vi "niWLAN - OPPO - 80211abgnGeneration(ref).vi"(0 "Rx Measurements Settings":T2 {"DSSS Data Rate (Mbps)" items=["1", "2", "5.5 CCK", "5.5 PBCC", "11 CCK", "11 PBCC", "22", "33"]; "OFDM Data Rate (Mbps)" items=["6", "9", "12", "18", "24", "36", "48", "54"]; "80211n PLCP Frame Format" items=["Mixed Format", "Greenfield Format"]; "Standard" items=["80211A/G/J/P OFDM", "80211B/G DSSS", "80211G DSSSOFDM", "80211N MIMOOFDM", "80211AC MIMOOFDM"]}, 5 "Without ACK ?":bool, 7 "Address String":string="00:90:4C:C5:12:38", 11 "error in":errorcluster) -> (4 "Cluster":T1, 15 "error out":errorcluster)   [LabVIEW 2010]
uses:
  <libdir>/resource/objmgr/niWLANGeneration.rc
  <vilib>/RF Toolkits/WLAN/generation/niWLANG Create Multiple Channel Waveform (IQ Complex Cluster).vi
  <vilib>/RF Toolkits/WLAN/generation/niWLANG Create Single Channel Waveform (IQ Complex Cluster).vi
  <vilib>/RF Toolkits/WLAN/generation/controls/wlanG version control.ctl
  TV/RW/Includes/WLAN - TV - RW - INC - Rx_PER_Wfm_Settings.ctl
panel:
  in  "Boolean":bool
  in  "Idle Time (With Ack)":dbl
  in  "file path":path
  # "Hardware Configuration"
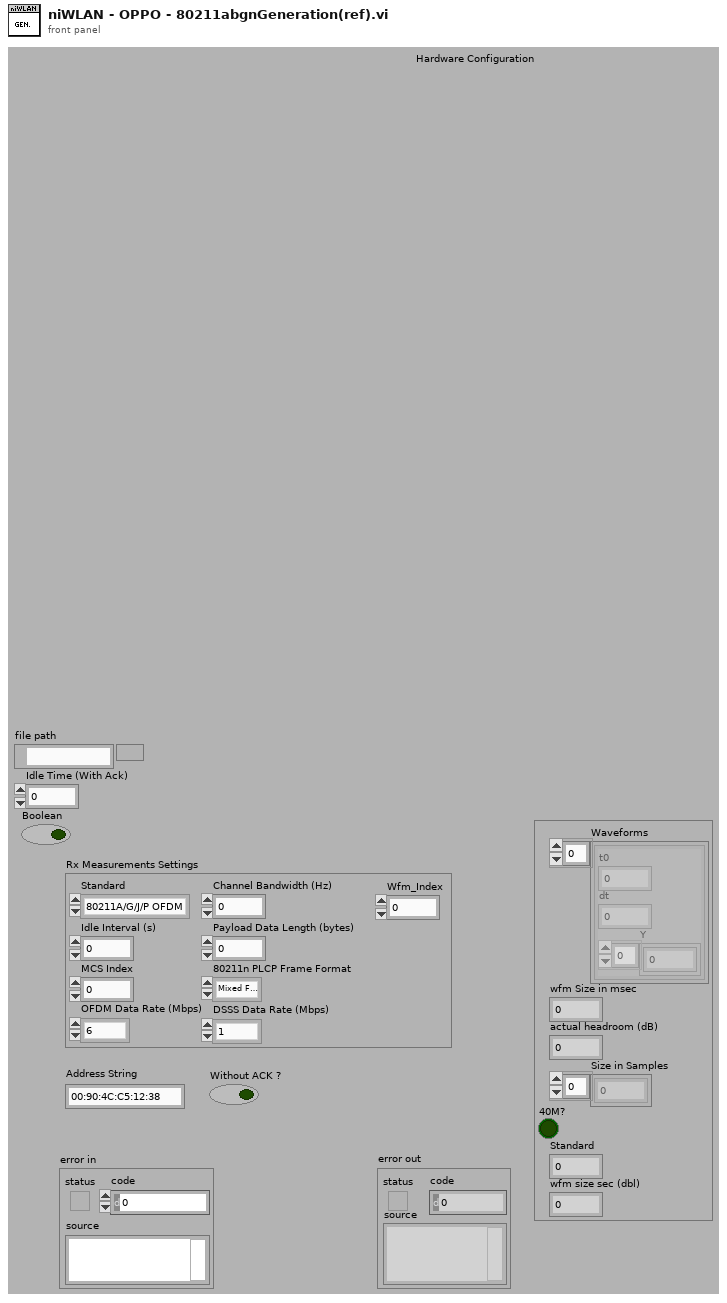
[diagram p1: front panel]
types:
  T1 = cluster{"Waveforms":cluster{"t0":dbl, "dt":dbl, "Y":cdb[]}[], "wfm Size in msec":i32, "actual headroom (dB)":dbl, "Size in Samples":i32[], "40M?":bool, "Standard ":i32, "wfm size sec (dbl)":dbl}
  T2 = typedef "WLAN - TV - RW - INC - Rx_PER_Wfm_Settings.ctl" = cluster{"Standard":i32, "Channel Bandwidth (Hz)":dbl, "Idle Interval (s)":dbl, "MCS Index":i32, "80211n PLCP Frame Format":i32, "Payload Data Length (bytes)":i32, "OFDM Data Rate (Mbps)":i32, "DSSS Data Rate (Mbps)":i32, "Wfm_Index":i32}
  T3 = typedef "wlanG version control.ctl" = i32
  T4 = typedef "wlanv1_generation refnum.ctl" = refnum<k20>
  T5 = typedef "wlanv1_Generation Refnum.ctl" = refnum<k20>
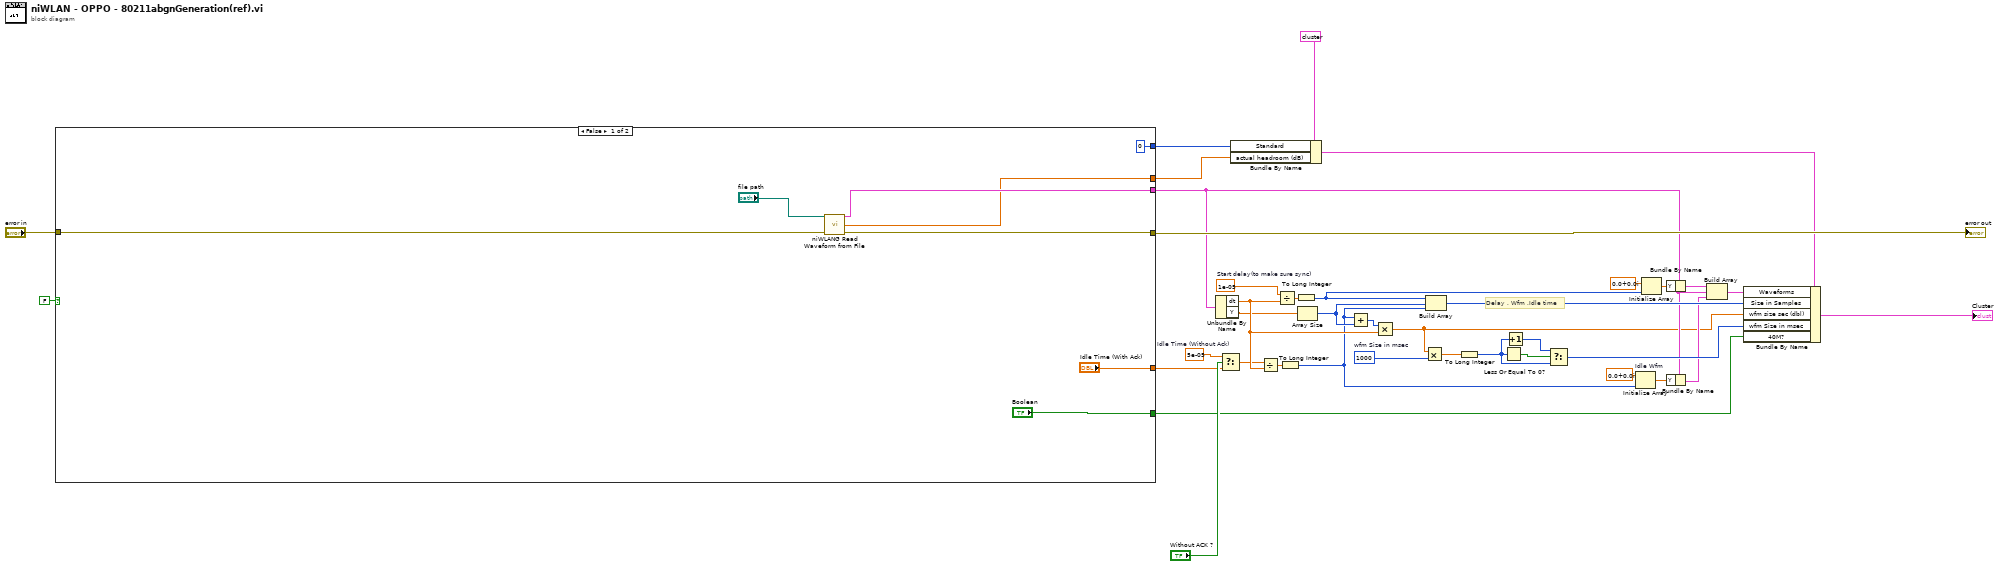
[diagram p0: block diagram]
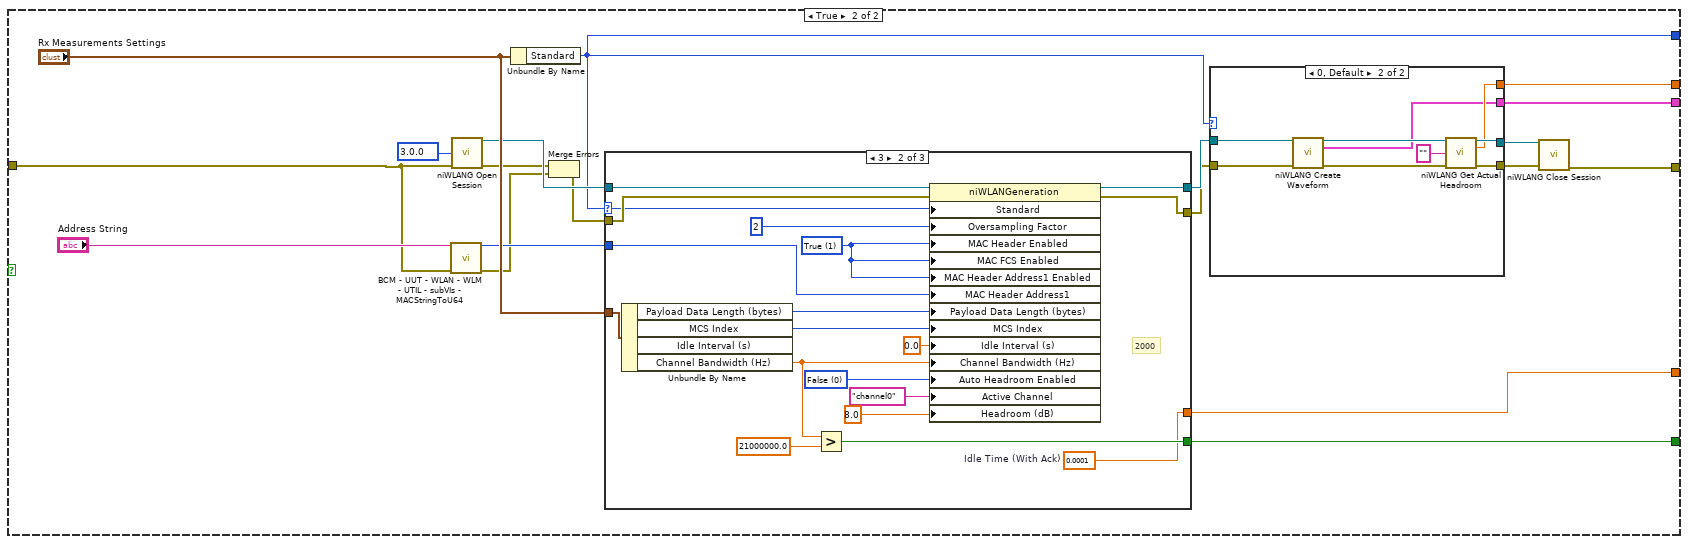
[diagram p2: hidden frame]
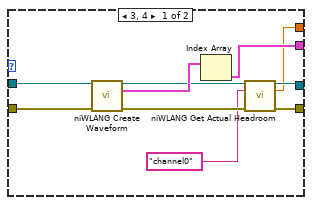
[diagram p3: hidden frame]
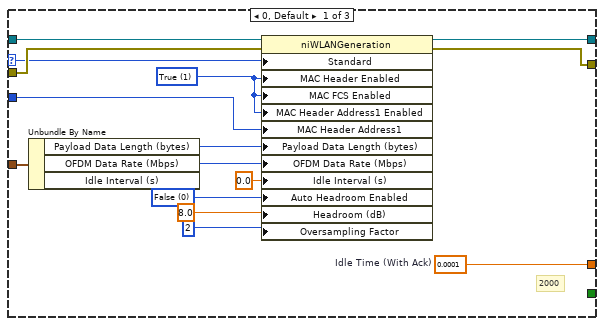
[diagram p4: hidden frame]
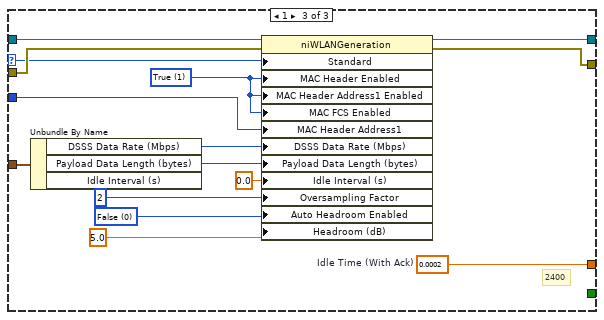
[diagram p5: hidden frame]
diagram:
  w16 = 1e-05  # Start delay(to make sure sync)
  w6 = 5e-05  # Idle Time (Without Ack)
  w15 = 1000  # wfm Size in msec
  # "Delay , Wfm ,Idle time"
  n1 = case shown="False" FALSE {
    tunnel: [w46 w64] -> w38
    tunnel: ["Boolean" w52] -> w25
    tunnel: [w45 w51] -> w18
    tunnel: [0 ("Standard") w50] -> w10
    tunnel: [w44 w49] -> w8
    tunnel: ["Idle Time (With Ack)" w48] -> w4
    tunnel: "error in" -> [w43 w47]
    frame False {
      n2 = call <vilib>:"niWLANG Read Waveform from File.vi"("file path"="file path", "error in"=w43) -> ("waveform"=w45:cluster{"t0":dbl, "dt":dbl, "Y":cdb[]}, "headroom (dB)"=w44:dbl, "error out"=w46:errorcluster)  [unwired: 9 in, 2 out]
    }
    frame True {
      w60 = T3 30000 items=["1.0.0"=10000, "2.0.0"=20000, "3.0.0"=30000] ("toolkit compatibility version")
      n3 = call "BCM - UUT - WLAN - WLM - UTIL - subVIs - MACStringToU64.vi"("Address String"="Address String", "error in"=w47) -> ("Address U64"=w62:u64, "error out"=w58:errorcluster)  [unwired: 12 in]
      n4 = call <vilib>:"niWLANG Open Session.vi"("toolkit compatibility version"=w60, "error in"=w47) -> ("niwlan generation session"=w61:T4, "error out"=w59:errorcluster)  [unwired: 11 in, 1 out]
      n5 = Unbundle By Name("Rx Measurements Settings") -> ("Standard"=w50:i32)
      n6 = Merge Errors(w59, w58) -> (w57:errorcluster)
      n7 = case shown="3" w50 {
        selector: w50 -> [w94 w113 w130]
        tunnel: w61 -> [w99 w117 w133]
        tunnel: w57 -> [w98 w114 w132]
        tunnel: [w97 w116 w131] -> w54
        tunnel: [w96 w115 w121] -> w53
        tunnel: w62 -> [w89 w106 w126]
        tunnel: "Rx Measurements Settings" -> [w87 w110 w122]
        tunnel: [_ w102 _] -> w52
        tunnel: [w85 w100 w119] -> w48
        frame 0, Default {
          w85 = 0.0001  # Idle Time (With Ack)
          w92 = 0 items=["False", "True"] ("Auto Headroom Enabled")
          w95 = 1 items=["False", "True"] ("MAC Header Enabled")
          # "2000"
          n8 = Unbundle By Name(w87) -> ("Payload Data Length (bytes)"=w90:i32, "OFDM Data Rate (Mbps)"=w93:i32)  [unwired: 1 out]
          n9 = property class="niWLANGeneration"(reference=w99, error in=w98, "Standard"=w94, "MAC Header Enabled"=w95, "MAC FCS Enabled"=w95, "MAC Header Address1 Enabled"=w95, "MAC Header Address1"=w89, "Payload Data Length (bytes)"=w90, "OFDM Data Rate (Mbps)"=w93, "Idle Interval (s)"=0.0, "Auto Headroom Enabled"=w92, "Headroom (dB)"=8.0, "Oversampling Factor"=2) -> (reference out=w97:T4, error out=w96:errorcluster)
        }
        frame 3 {
          w100 = 0.0001  # Idle Time (With Ack)
          w109 = 0 items=["False", "True"] ("Auto Headroom Enabled")
          w118 = 1 items=["False", "True"] ("MAC Header Enabled")
          # "2000"
          n10 = Unbundle By Name(w110) -> ("Payload Data Length (bytes)"=w112:i32, "MCS Index"=w111:i32, "Channel Bandwidth (Hz)"=w105:dbl)  [unwired: 1 out]
          n11 = Greater?(x=w105, y=21000000.0) -> (0:w102:bool)
          n12 = property class="niWLANGeneration"(reference=w117, error in=w114, "Standard"=w113, "Oversampling Factor"=2, "MAC Header Enabled"=w118, "MAC FCS Enabled"=w118, "MAC Header Address1 Enabled"=w118, "MAC Header Address1"=w106, "Payload Data Length (bytes)"=w112, "MCS Index"=w111, "Idle Interval (s)"=0.0, "Channel Bandwidth (Hz)"=w105, "Auto Headroom Enabled"=w109, "Active Channel"="channel0", "Headroom (dB)"=8.0) -> (reference out=w116:T4, error out=w115:errorcluster)
        }
        frame 1 {
          w119 = 0.0002  # Idle Time (With Ack)
          w124 = 0 items=["False", "True"] ("Auto Headroom Enabled")
          w129 = 1 items=["False", "True"] ("OFDM Demod Enabled")
          # "2400"
          n13 = Unbundle By Name(w122) -> ("DSSS Data Rate (Mbps)"=w128:i32, "Payload Data Length (bytes)"=w127:i32)  [unwired: 1 out]
          n14 = property class="niWLANGeneration"(reference=w133, error in=w132, "Standard"=w130, "MAC Header Enabled"=w129, "MAC Header Address1 Enabled"=w129, "MAC FCS Enabled"=w129, "MAC Header Address1"=w126, "DSSS Data Rate (Mbps)"=w128, "Payload Data Length (bytes)"=w127, "Idle Interval (s)"=0.0, "Oversampling Factor"=2, "Auto Headroom Enabled"=w124, "Headroom (dB)"=5.0) -> (reference out=w131:T4, error out=w121:errorcluster)
        }
      }
      n15 = case shown="0, Default" w50 {
        tunnel: [w70 w81] -> w55
        tunnel: w54 -> [w74 w84]
        tunnel: w53 -> [w75 w83]
        tunnel: [w68 w80] -> w56
        tunnel: [w72 w76] -> w51
        tunnel: [w66 w78] -> w49
        frame 3, 4 {
          n16 = call-poly <vilib>:"niWLANG Create Waveform.vi"("niwlan generation session"=w74, "error in"=w75) -> ("niwlan generation session out"=w71:T4, "output waveform"=w73:cluster{"t0":dbl, "dt":dbl, "Y":cdb[]}[], "error out"=w69:errorcluster)  [unwired: 10 in, 1 out]
          n17 = Index Array(array=w73) -> (element=w72:cluster{"t0":dbl, "dt":dbl, "Y":cdb[]})  [unwired: 1 in]
          n18 = call <vilib>:"niWLANG Get Actual Headroom.vi"("niwlan generation session"=w71, "active channel"="channel0", "error in"=w69) -> ("niwlan generation session out"=w70:T5, "actual headroom (dB)"=w66:dbl, "error out"=w68:errorcluster)  [unwired: 10 in]
        }
        frame 0, Default {
          n19 = call-poly <vilib>:"niWLANG Create Waveform.vi"("niwlan generation session"=w84, "error in"=w83) -> ("niwlan generation session out"=w82:T4, "output waveform"=w76:cluster{"t0":dbl, "dt":dbl, "Y":cdb[]}, "error out"=w79:errorcluster)  [unwired: 10 in, 1 out]
          n20 = call <vilib>:"niWLANG Get Actual Headroom.vi"("niwlan generation session"=w82, "active channel"="", "error in"=w79) -> ("niwlan generation session out"=w81:T5, "actual headroom (dB)"=w78:dbl, "error out"=w80:errorcluster)  [unwired: 10 in]
        }
      }
      n21 = call <vilib>:"niWLANG Close Session.vi"("niwlan generation session"=w55, "error in"=w56) -> ("error out"=w64:errorcluster)  [unwired: 13 in]
    }
  }
  "error out" <- w38
  n22 = Unbundle By Name(w18) -> ("dt"=w17:dbl, "Y"=w11:cdb[])
  n23 = Select(t=w6, s="Without ACK ?", f=w4) -> (s? t:f=w5:dbl)
  n24 = Bundle By Name(cluster=T1 {"Waveforms"=[{"t0"=0.0, "dt"=1.25e-08, "Y"=array[800 elements]}, {"t0"=0.0, "dt"=1.25e-08, "Y"=array[85448 elements]}], "wfm Size in msec"=1, "actual headroom (dB)"=0.0, "Size in Samples"=[10000000, 0], "40M?"=TRUE, "Standard "=3, "wfm size sec (dbl)"=0.0} ("Cluster"), "Standard"=w10, "actual headroom (dB)"=w8) -> (w9:T1)
  n25 = Divide(x=w5, y=w17) -> (x/y=w20:dbl)
  n26 = Divide(x=w16, y=w17) -> (x/y=w32:dbl)
  n27 = To Long Integer(number=w20) -> (32bit integer=w7:i32)
  n28 = To Long Integer(number=w32) -> (32bit integer=w31:i32)
  n29 = Array Size(array=w11) -> (size(s)=w21:i32)
  n30 = Add(x=w7, y=w21) -> (x+y=w19:i32)
  n31 = Multiply(x=w19, y=w17) -> (x*y=w13:dbl)
  n32 = Multiply(x=w13, y=w15) -> (x*y=w14:dbl)
  n33 = Build Array(w31, w21, w7) -> (w27:i32[])
  n34 = To Long Integer(number=w14) -> (32bit integer=w34:i32)
  n35 = Less Or Equal To 0?(x=w34) -> (x <= 0?=w35:bool)
  n36 = Increment(x=w34) -> (x+1=w33:i32)
  n37 = Select(t=w33, s=w35, f=w34) -> (s? t:f=w26:i32)
  n38 = Initialize Array "Idle Wfm"(cdb 0.0+0.0i ("element"), w7) -> (w23:cdb[])
  n39 = Initialize Array(cdb 0.0+0.0i ("element"), w31) -> (w30:cdb[])
  n40 = Bundle By Name(cluster=w18, "Y"=w30) -> (w29:cluster{"t0":dbl, "dt":dbl, "Y":cdb[]})
  n41 = Bundle By Name(cluster=w18, "Y"=w23) -> (w22:cluster{"t0":dbl, "dt":dbl, "Y":cdb[]})
  n42 = Build Array(w29, w18, w22) -> (w28:cluster{"t0":dbl, "dt":dbl, "Y":cdb[]}[])
  n43 = Bundle By Name(cluster=w9, "Waveforms"=w28, "Size in Samples"=w27, "wfm size sec (dbl)"=w13, "wfm Size in msec"=w26, "40M?"=w25) -> (→"Cluster":T1)
